vi "Trav_pos_for_Email.vi"() -> (0 "String":string)   [LabVIEW 2011]
uses:
  Controls/Overhead.ctl
  Globals/Trav_pos_global.vi
  Globals/Meas_global.vi
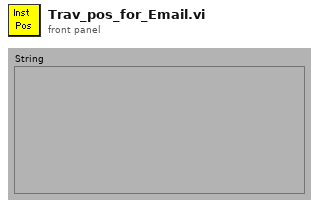
[diagram p1: front panel]
types:
  T1 = typedef "Overhead.ctl" = enum16{"Update total times", "Read Current Overhead", "Re Scale totals to 3 hrs", "Initialise totals to 3hr"}
  T2 = typedef "Tunnel_Coordinates.ctl" = enum16{"Work in Tunnel Coordinates", "Work in Model Coordinates"}
  T3 = typedef "Traverse_cluster.ctl" = cluster{"Start X":dbl, "Start Y":dbl, "Start Z":dbl, "End X":dbl, "End Y":dbl, "End Z":dbl, "No. of pts.":i32, "Spacing":T4, "Filename":path, "Tunnel Speed":dbl, "Averaging time (min)":dbl, "Extra Commands":string, "Specific Arguments":string, "Emission Rate (l/min)":dbl, "Trace Gas Concentration (%)":dbl, "Density Ratio":string, "Comments":string, "Row No":i32, "Row Type Selector":T5, "Completion time":string, "Row Duration (mins)":dbl, "No. of Valid pts.":i32, "Meas Setup File":string}
  T4 = typedef "Spacing.ctl" = enum16{"Linear", "Log", "Gauss", "Specified", "N/A"}
  T5 = typedef "Multi_run_mode.ctl" = enum16{"Move Traverse Only", "Set Tunnel Speed Only", "Set Source Only", "Set Measurement Conditions", "Single Measurement", "Vertical Profile", "Lateral Profile", "Longitudinal Profile", "Explore Volume", "Multi-Axis Profile", "Auto Calibrate", "Meas Fast FID Bkgnd", "Check Beam Power", "Scanning Valve Measurement", "Run VI Named:", "Set ADAM Ch", "Wait (minutes)", "Send Message", "Synchronize With:", "Fall Back to this Row", "Turn Off Row Repeating", "Blank Row"}
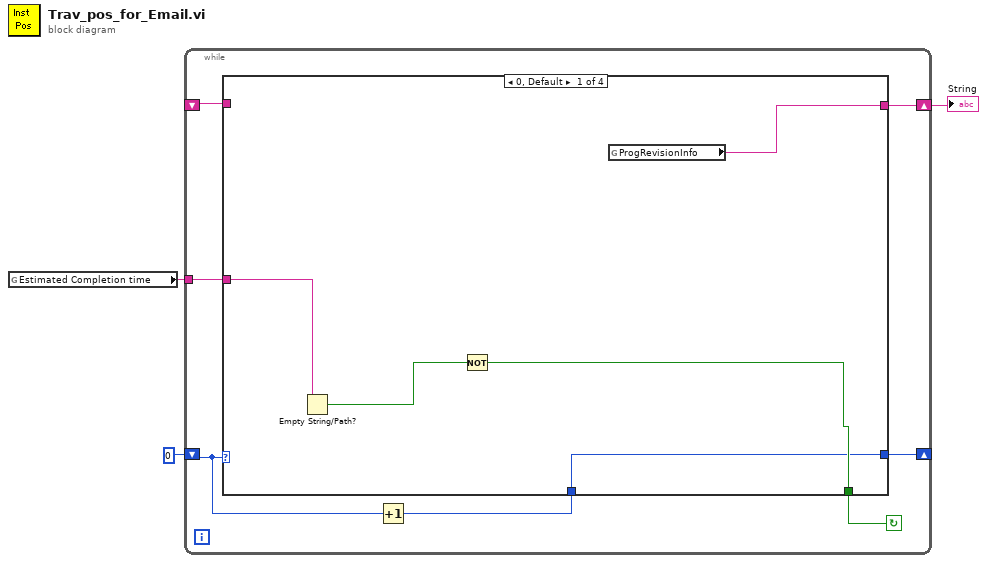
[diagram p0: block diagram]
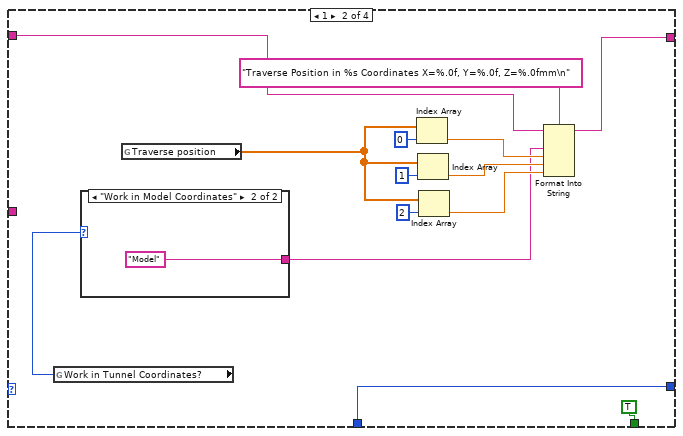
[diagram p2: hidden frame]
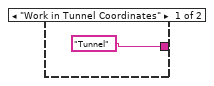
[diagram p3: hidden frame]
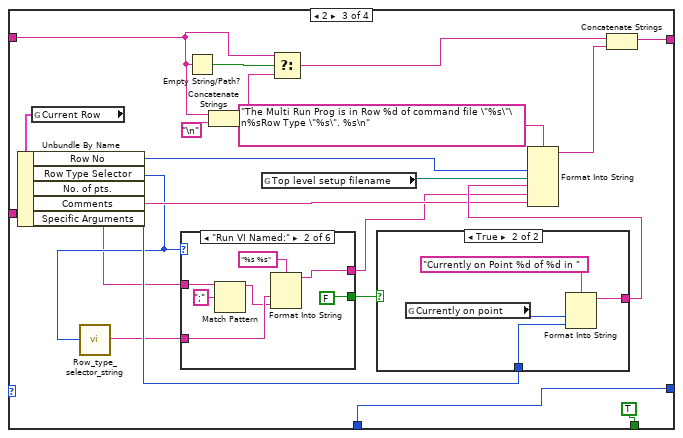
[diagram p4: hidden frame]
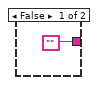
[diagram p5: hidden frame]
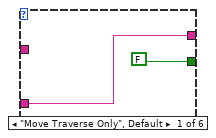
[diagram p6: hidden frame]
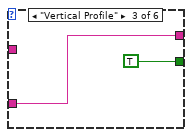
[diagram p7: hidden frame]
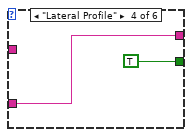
[diagram p8: hidden frame]
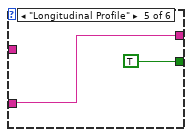
[diagram p9: hidden frame]
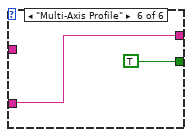
[diagram p10: hidden frame]
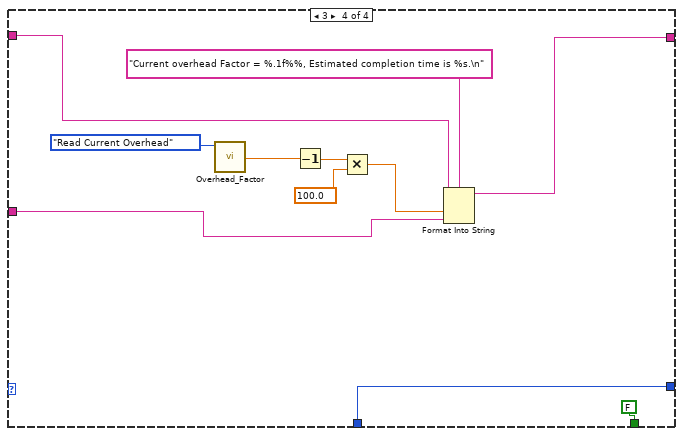
[diagram p11: hidden frame]
diagram:
  n1 = global read "Trav_pos_global.vi" "Estimated Completion time"() -> (w1:string)
  n2 = while {
    shift-left: _ -> [w5]
    shift-right: [w7] -> w2
    shift-left: 0 -> [w10]
    shift-right: [w9] -> _
    tunnel: w1 -> [w4]
    stop <- w6 continue-if-true
    n3 = Increment(x=w10) -> (x+1=w8:i32)
    n4 = case shown="0, Default" w10 {
      tunnel: [w12 w29 w46 w84] -> w9
      tunnel: w8 -> [w12 w29 w46 w84]
      tunnel: [w11 w20 w52 w76] -> w7
      tunnel: [w13 TRUE TRUE FALSE] -> w6
      tunnel: w5 -> [_ w21 w43 w77]
      tunnel: w4 -> [w15 _ _ w75]
      frame 0, Default {
        n5 = Empty String/Path?(string/path=w15) -> (empty?=w14:bool)
        n6 = Not(x=w14) -> (.not. x?=w13:bool)
        n7 = global read "Meas_global.vi" "ProgRevisionInfo"() -> (w11:string)
      }
      frame 1 {
        n8 = global read "Trav_pos_global.vi" "Work in Tunnel Coordinates?"() -> (w19:T2)
        n9 = case shown="\"Work in Model Coordinates\"" w19 {
          tunnel: ["Tunnel" "Model"] -> w17
          frame "Work in Tunnel Coordinates" {
          }
          frame "Work in Model Coordinates" {
          }
        }
        n10 = global read "Trav_pos_global.vi" "Traverse position"() -> (w16:dbl[])
        n11 = Index Array(array=w16, index=0) -> (element=w18:dbl)
        n12 = Index Array(array=w16, index=1) -> (element=w23:dbl)
        n13 = Index Array(array=w16, index=2) -> (element=w22:dbl)
        n14 = Format Into String(format string="Traverse Position in %s Coordinates X=%.0f, Y=%.0f, Z=%.0fmm\n" ("Format String"), initial string=w21, w17, w18, w23, w22) -> (resulting string=w20:string)  [unwired: 1 in, 1 out]
      }
      frame 2 {
        n15 = global read "Trav_pos_global.vi" "Current Row"() -> (w37:T3)
        n16 = Unbundle By Name(w37) -> ("Row No"=w51:i32, "Row Type Selector"=w35:T5, "No. of pts."=w49:i32, "Comments"=w36:string, "Specific Arguments"=w32:string)
        n17 = call "Row_type_selector_string.vi"("Mode"=w35) -> ("Output string"=w34:string)
        n18 = case shown="\"Run VI Named:\"" w35 {
          tunnel: [FALSE FALSE TRUE TRUE TRUE TRUE] -> w50
          tunnel: w34 -> [w58 w65 w67 w69 w71 w73]
          tunnel: [w58 w63 w67 w69 w71 w73] -> w33
          tunnel: w32 -> [_ w61 _ _ _ _]
          frame "Move Traverse Only", Default {
          }
          frame "Run VI Named:" {
            n19 = Match Pattern(string=w61, regular expression=";") -> (before substring=w60:string)  [unwired: 4 out]
            n20 = Format Into String(format string="%s %s" ("Format String"), w65, w60) -> (resulting string=w63:string)  [unwired: 2 in, 1 out]
          }
          frame "Vertical Profile" {
          }
          frame "Lateral Profile" {
          }
          frame "Longitudinal Profile" {
          }
          frame "Multi-Axis Profile" {
          }
        }
        n21 = Empty String/Path?(string/path=w43) -> (empty?=w45:bool)
        n22 = Concatenate Strings(w43, "\n") -> (w44:string)
        n23 = global read "Trav_pos_global.vi" "Top level setup filename"() -> (w40:path)
        n24 = Select(t=w43, s=w45, f=w44) -> (s? t:f=w42:string)
        n25 = case shown="True" w50 {
          tunnel: w49 -> [_ w56]
          tunnel: ["" w54] -> w39
          frame False {
          }
          frame True {
            n26 = global read "Trav_pos_global.vi" "Currently on point"() -> (w57:i32)
            n27 = Format Into String(format string="Currently on Point %d of %d in " ("Format String"), w57, w56) -> (resulting string=w54:string)  [unwired: 2 in, 1 out]
          }
        }
        n28 = Format Into String(format string="The Multi Run Prog is in Row %d of command file \"%s\"\n%sRow Type \"%s\". %s\n" ("Format String"), w51, w40, w39, w33, w36) -> (resulting string=w38:string)  [unwired: 2 in, 1 out]
        n29 = Concatenate Strings(w42, w38) -> (w52:string)
      }
      frame 3 {
        n30 = call "Overhead_Factor.vi"("Mode"=Overhead."Read Current Overhead") -> ("Current Overhead Factor"=w82:dbl)  [unwired: 3 in]
        n31 = Decrement(x=w82) -> (x-1=w81:dbl)
        n32 = Multiply(x=w81, y=100.0) -> (x*y=w79:dbl)
        n33 = Format Into String(format string="Current overhead Factor = %.1f%%, Estimated completion time is %s.\n" ("Format String"), initial string=w77, w79, w75) -> (resulting string=w76:string)  [unwired: 1 in, 1 out]
      }
    }
  }
  "String" <- w2
